vi "Set Initialization Data - Spectro Acq.vi"(8 "error in":errorcluster, 11 "UI SmarAct in":refnum<class "UI SmarAct.lvclass">) -> (0 "error out":errorcluster, 3 "UI SmarAct out":refnum<class "UI SmarAct.lvclass">)   [LabVIEW 2024, in "UI SmarAct.lvclass"]
doc: "In this VI you can set the initialization data of a statically-linked subWorker."
uses:
  UI SmarAct.lvclass
  Spectro Acquisition/Initialization Data.ctl
  Spectro Acquisition/Response Cases.ctl
  Data Queue.ctl
  UI SmarAct.lvclass/UI SmarAct.ctl
  Spectro Acquisition/Spectro Acquisition.lvclass
  C:/Program Files (x86)/National Instruments/LabVIEW 2024/vi.lib/addons/_Workers/Library/Classes/Worker/Worker.lvclass
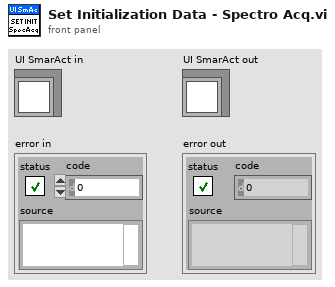
[diagram p1: front panel]
types:
  T1 = typedef "Spectro Acquisition.lvclass/Initialization Data.ctl" = cluster{"Data Spectro":T2, "Data Queue":T3}
  T2 = typedef "Spectro Acquisition.lvclass/Response Cases.ctl" = cluster{"Placeholder - Can be deleted":string, "Wrapper Spectro":u32, "Calib en intensité":dbl[], "Calib?":bool}
  T3 = typedef "UI SmarAct.lvclass/Data Queue.ctl" = cluster{"Queue Data":refnum<queue>}
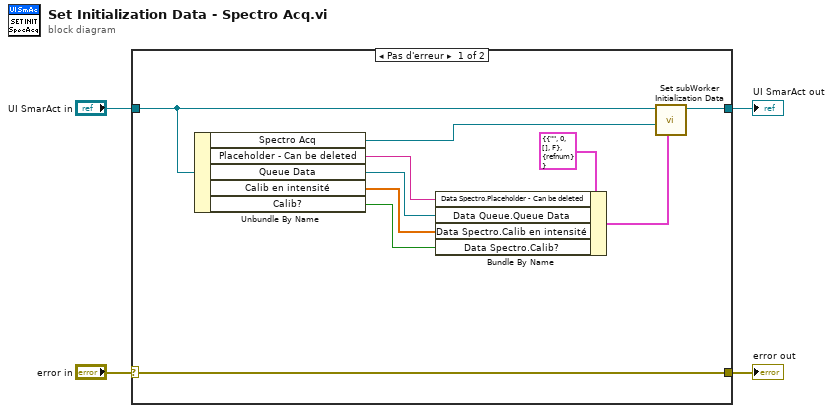
[diagram p0: block diagram]
diagram:
  n1 = case shown="Pas d'erreur" "error in" {
    selector: "error in" -> [w14 w16]
    tunnel: [w14 w16] -> w3
    tunnel: [w12 w15] -> w2
    tunnel: "UI SmarAct in" -> [w11 w15]
    frame No Error {
      n2 = Unbundle By Name(w11) -> ("Spectro Acq"=w13:refnum<class "Spectro Acquisition.lvclass">, "Placeholder - Can be deleted"=w8:string, "Queue Data"=w7:refnum<queue>, "Calib en intensité"=w6:dbl[], "Calib?"=w5:bool)
      n3 = Bundle By Name(cluster=T1 {"Data Spectro"={"Placeholder - Can be deleted"="", "Wrapper Spectro"=0, "Calib en intensité"=[], "Calib?"=FALSE}, "Data Queue"={"Queue Data"=refnum}} ("Initialization Data"), "Data Spectro.Placeholder - Can be deleted"=w8, "Data Queue.Queue Data"=w7, "Data Spectro.Calib en intensité"=w6, "Data Spectro.Calib?"=w5) -> (w9:T1)
      n4 = call-dynamic "Set subWorker Initialization Data.vi"("Initialization Data"=w9, "subWorker"=w13, "Worker"=w11) -> ("Worker out"=w12:refnum<class "UI SmarAct.lvclass">)  [unwired: 8 in]
    }
    frame Error {
    }
  }
  "error out" <- w3
  "UI SmarAct out" <- w2
